vi "Main.vi"() -> ()   [LabVIEW 2020]
panel:
  out "appended path 3":path
  out "appended path 2":path
  out "appended path":path
  in  "Error in":errorcluster
  out "error out":errorcluster
  out "x+y":dbl format="%_9g"
  in  "Stop":bool
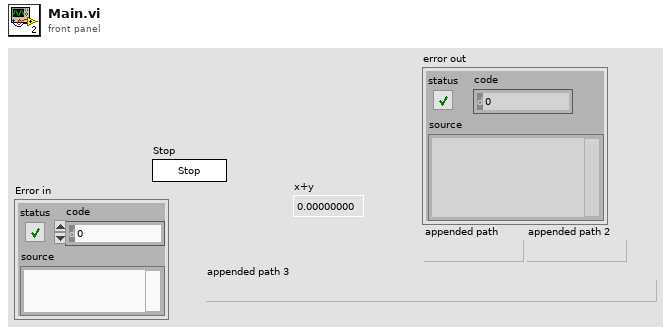
[diagram p1: front panel]
types:
  T1 = enum16{"open", "replace", "create", "open or create", "replace or create", "replace or create with confirmation"}
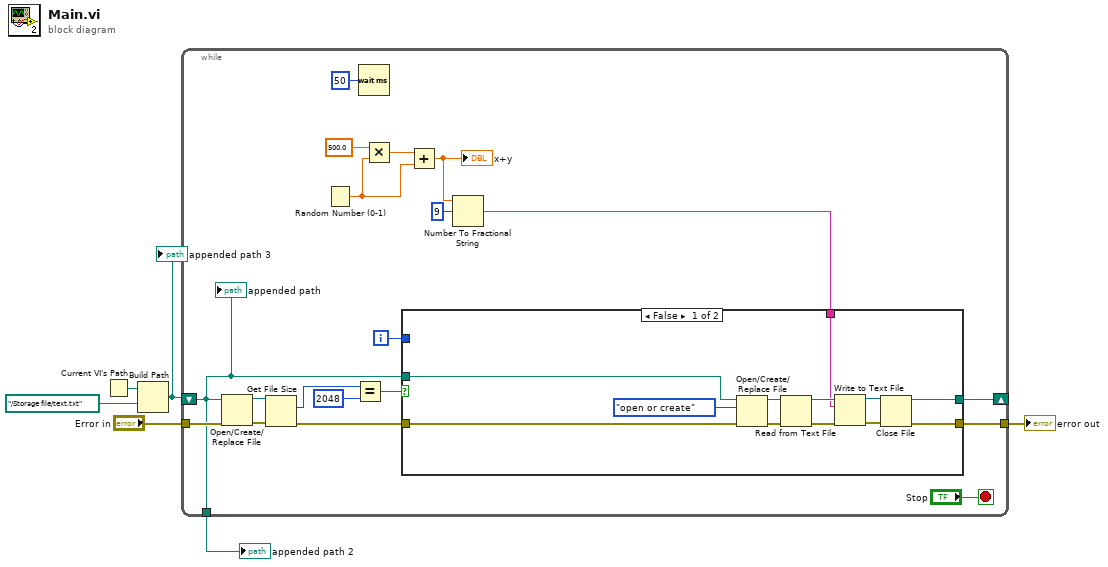
[diagram p0: block diagram]
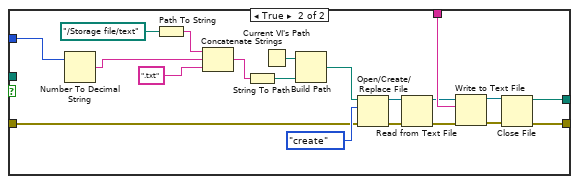
[diagram p2: hidden frame]
diagram:
  n1 = Current VI's Path() -> (path=w4:path)
  n2 = Build Path(base path=w4, name or relative path=path "../Storage file/text.txt") -> (appended path=w1:path)
  "appended path 3" <- w1
  n3 = while {
    tunnel: [w17] -> w6
    tunnel: "Error in" -> [w10]
    shift-right: [w16] -> _
    shift-left: w1 -> [w7]
    tunnel: [w7] -> w2
    i -> [w11]
    stop <- "Stop" stop-if-true
    n4 = Open/Create/Replace File(file path (use dialog)=w7, error in=w10) -> (refnum out=w9:refnum<file>, error out=w8:errorcluster)  [unwired: 4 in, 1 out]
    n5 = Get File Size(file=w9, error in=w8) -> (size (in bytes)=w14:i64, 0:w12:errorcluster)  [unwired: 1 out]
    n6 = Random Number (0-1)() -> (number: 0 to 1=w21:dbl)
    n7 = Equal?(x=w14, y=i64 2048) -> (x = y?=w15:bool)
    n8 = Wait (ms)(milliseconds to wait=u32 50) -> ()  [unwired: 1 out]
    n9 = Multiply(x=500.0, y=w21) -> (x*y=w22:dbl)
    n10 = Add(x=w22, y=w21) -> (x+y=w20:dbl)
    "x+y" <- w20
    n11 = Number To Fractional String(number=w20, width (-)=i16 9) -> (F-format string=w18:string)  [unwired: 2 in]
    n12 = case shown="False" w15 {
      tunnel: w18 -> [w28 w54]
      tunnel: [w29 w53] -> w17
      tunnel: w12 -> [w30 w52]
      tunnel: [w27 w47] -> w16
      tunnel: w11 -> [_ w42]
      tunnel: w7 -> [w26 _]
      frame False {
        n13 = Open/Create/Replace File(file path (use dialog)=w26, error in=w30, operation (0:open)=T1."open or create") -> (refnum out=w34:refnum<file>, error out=w32:errorcluster)  [unwired: 3 in, 1 out]
        n14 = Read from Text File(file (use dialog)=w34, error in=w32) -> (refnum out=w33:refnum<file>, error out=w31:errorcluster)  [unwired: 2 in, 2 out]
        n15 = Write to Text File(file (use dialog)=w33, text=w28, error in=w31) -> (refnum out=w36:refnum<file>, error out=w35:errorcluster)  [unwired: 1 in, 1 out]
        n16 = Close File(refnum=w36, error in=w35) -> (path=w27:path, error out=w29:errorcluster)
      }
      frame True {
        n17 = Number To Decimal String(number=w42) -> (decimal integer string=w41:string)  [unwired: 1 in]
        n18 = Path To String(path=path "../Storage file/text" ("name or relative path")) -> (string=w43:string)
        n19 = Concatenate Strings(w43, w41, ".txt" ("string")) -> (w38:string)
        n20 = String To Path(string=w38) -> (path=w39:path)
        n21 = Current VI's Path() -> (path=w46:path)
        n22 = Build Path(base path=w46, name or relative path=w39) -> (appended path=w45:path)
        n23 = Open/Create/Replace File(file path (use dialog)=w45, error in=w52, operation (0:open)=T1."create") -> (refnum out=w51:refnum<file>, error out=w49:errorcluster)  [unwired: 3 in, 1 out]
        n24 = Read from Text File(file (use dialog)=w51, error in=w49) -> (refnum out=w50:refnum<file>, error out=w48:errorcluster)  [unwired: 2 in, 2 out]
        n25 = Write to Text File(file (use dialog)=w50, text=w54, error in=w48) -> (refnum out=w56:refnum<file>, error out=w55:errorcluster)  [unwired: 1 in, 1 out]
        n26 = Close File(refnum=w56, error in=w55) -> (path=w47:path, error out=w53:errorcluster)
      }
    }
    "appended path" <- w7
  }
  "error out" <- w6
  "appended path 2" <- w2
